vi "comms_Serial_Send_Com.vi"(8 "error in":errorcluster, 9 "Buffer Clear?":bool, 10 "Command":string, 11 "VISA resource in":refnum<visa-resource-name>) -> (0 "error out":errorcluster, 2 "Response":string, 3 "VISA resource Out":refnum<visa-resource-name>)   [LabVIEW 2018]
panel:
  out "cleared data":string
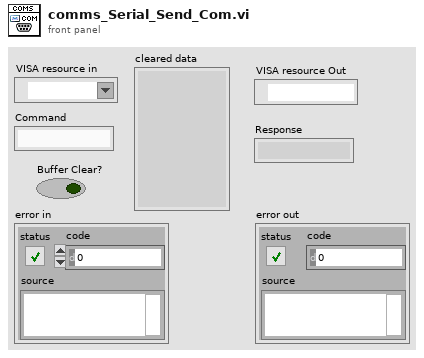
[diagram p1: front panel]
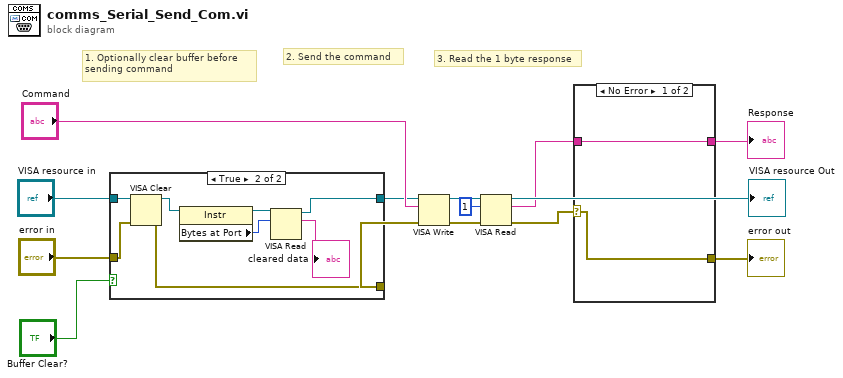
[diagram p0: block diagram]
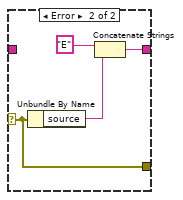
[diagram p2: hidden frame]
diagram:
  # "3. Read the 1 byte response"
  # "2. Send the command"
  # "1. Optionally clear buffer before \nsending command"
  n1 = case shown="True" "Buffer Clear?" {
    tunnel: "VISA resource in" -> [w16 w24]
    tunnel: [w16 w18] -> w6
    tunnel: "error in" -> [w15 w23]
    tunnel: [w15 w22] -> w9
    frame False {
    }
    frame True {
      n2 = VISA Clear(VISA resource name=w24, error in (no error)=w23) -> (VISA resource name out=w19:refnum<visa-resource-name>, error out=w22:errorcluster)
      n3 = property class="Instr"(reference=w19) -> (reference out=w20:refnum<visa-resource-name>, "Bytes at Port"=w21:u32)  [unwired: 1 in, 1 out]
      n4 = VISA Read(VISA resource name=w20, byte count=w21) -> (VISA resource name out=w18:refnum<visa-resource-name>, read buffer=→"cleared data":string)  [unwired: 1 in, 2 out]
    }
  }
  n5 = VISA Write(VISA resource name=w6, write buffer="Command", error in (no error)=w9) -> (VISA resource name out=w5:refnum<visa-resource-name>, error out=w8:errorcluster)  [unwired: 1 out]
  n6 = VISA Read(VISA resource name=w5, byte count=u32 1, error in (no error)=w8) -> (VISA resource name out=→"VISA resource Out":refnum<visa-resource-name>, read buffer=w2:string, error out=w4:errorcluster)  [unwired: 1 out]
  n7 = case shown="No Error" w4 {
    selector: w4 -> [w26 w30]
    tunnel: [w26 w30] -> w3
    tunnel: w2 -> [w25 _]
    tunnel: [w25 w29] -> w1
    frame No Error {
    }
    frame Error {
      n8 = Unbundle By Name(w30) -> ("source"=w28:string)
      n9 = Concatenate Strings("E", w28) -> (w29:string)
    }
  }
  "error out" <- w3
  "Response" <- w1
